vi "Update Config.vi"(8 "error in":errorcluster, 10 "a":dbl) -> (0 "error out":errorcluster)   [LabVIEW 2020, in "CML UI.lvlib" / "Configuration.lvclass"]
doc: "Update a configuration value externally.\n____\nPeloton Config 2.0.0.9\nCopyright (c) 2024, Peloton"
uses:
  Configuration.lvclass
  Configuration.lvclass/Configuration.ctl
  <vilib>/Peloton/Peloton Config/DCFG Framework/Peloton_lib_DCFG Framework.lvlib
  CML UI.lvlib
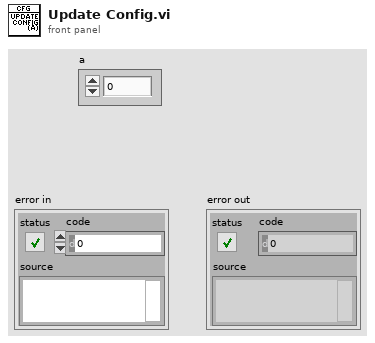
[diagram p1: front panel]
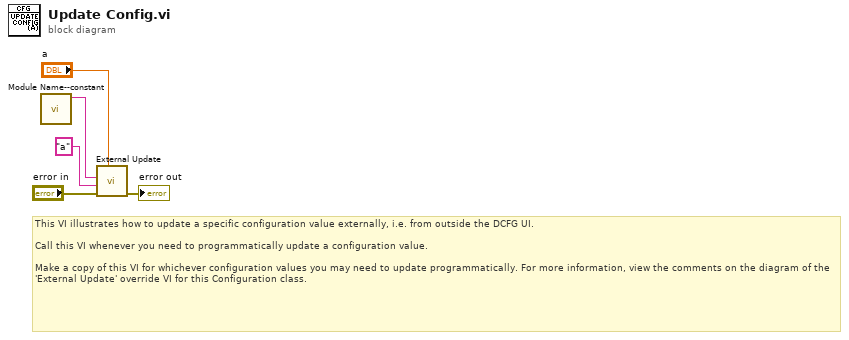
[diagram p0: block diagram]
diagram:
  # "This VI illustrates how to update a specific configuration value externally, i.e. from outside the DCFG UI.\n\nCall this VI whenever you need to programmatically update a configuration value.\n\nMake a copy of this VI for whichever configuration values you may need to update programmatically. For more information, view the comments on the diagram of the 'External Update' override VI for this Configuration class."
  n1 = call "Module Name--constant.vi"() -> ("Module Name"=w2:string)  [unwired: 11 in]
  n2 = call <vilib>:"External Update.vi"("Value"="a", "error in"="error in", "Parameter"="a", "Config Name"=w2) -> ("error out"=→"error out":errorcluster)  [unwired: 6 in, 1 out]
